vi "Caller VI_ApplyLibIconOverlayToVIIcon.vi"(4 "External User Layer":refnum<class "Layer.lvclass">[](array[class]), 6 "Add Ext User Layer? (F)":bool, 7 "Lib Refnum":refnum<vi>, 8 "Don't Consider Curr VI Icon? (F)":bool, 9 "Overlay Image":T1={"image type"=0, "image depth"=0, "image"=[], "mask"=[], "colors"=[], "Rectangle"={"left"=0, "top"=0, "right"=32, "bottom"=32}}, 10 "Overlay Provided?":bool, 11 "VI Refnum":refnum<vi>) -> (0 "Error Code Out":i32)   [LabVIEW 2021]
uses:
  <vilib>/picture/picture.llb/imagedata.ctl
  vi.lib/LabVIEW Icon API/lv_icon/Classes/Layer/Layer.lvclass
  vi.lib/LabVIEW Icon API/lv_icon/Classes/Icon/Icon.lvclass
  TypeDefs/Cluster_Layer Data.ctl
  TypeDefs/Cluster_Path&Icon.ctl
  vi.lib/LabVIEW Icon API/lv_icon/lv_icon.lvlib
  vi.lib/LabVIEW Icon API/lv_icon/Classes/Icon Framework/Icon Framework.lvclass
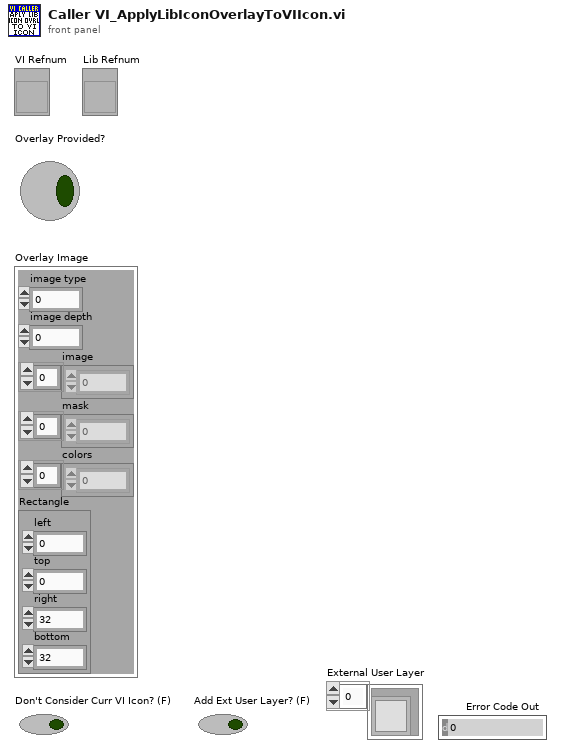
[diagram p1: front panel]
types:
  T1 = typedef "imagedata.ctl" = cluster{"image type":i32, "image depth":i32, "image":u8[], "mask":u8[], "colors":u32[], "Rectangle":cluster{"left":i16, "top":i16, "right":i16, "bottom":i16}}
  T2 = typedef "Cluster_Path&Icon.ctl" = cluster{"Rectangle":cluster{"left":i16, "top":i16, "right":i16, "bottom":i16}, "Path":path, "Image":picture, "Filter":string, "FileName":string}
  T3 = typedef "Cluster_Layer Data.ctl" = cluster{"LayerIcon":picture, "LayerName":string, "Opacity":u8, "Visibility?":bool}
  T4 = typedef "Cluster_INI Data.ctl" = cluster{"Show Layer Tab?":bool, "Show Terminals?":bool, "Text":cluster{"Font":T5, "Alignment":T6, "Size":T7}, "3rd party Templates":cluster{"Store 3rd party Templates?":bool, "Folder Name":string}, "Merge user layers on commit":bool, "Body Text":T8, "Fill Color":T9, "Edge Color":T9, "Tab":u16, "Tool":T10, "Disable Layers?":bool}
  T5 = typedef "Font.ctl" = string
  T6 = typedef "Alignment.ctl" = u16
  T7 = typedef "Num_Font Size.ctl" = u8
  T8 = typedef "Cluster_BodyText.ctl" = cluster{"Line 1 text":string, "Line 2 text":string, "Line 3 text":string, "Line 4 text":string, "Line 1 color":u32, "Line 2 color":u32, "Line 3 color":u32, "Line 4 color":u32, "Body Text Spec":cluster{"Font":T5, "Alignment":T6, "Size":u8}, "Center text vertically":bool, "Capitalize Text":bool}
  T9 = typedef "IEColor.ctl" = u32
  T10 = typedef "Cluster_Button Draw Tools.ctl" = enum32{"Pencil", "Line", "Dropper", "Fill", "Rectangle", "Filled Rectangle", "Ellipse", "Filled Ellipse", "Eraser", "Text", "Select", "Move"}
  T11 = typedef "LabVIEW Icon Stored Information.ctl" = cluster{"Text Visible?":bool, "Text Opacity":u8, "Templ Visible?":bool, "Templ Opacity":u8, "Relative Path from 1 to 2":path, "Image":picture, "All User Layers":refnum<class "Layer.lvclass">[], "Body Text":T8}
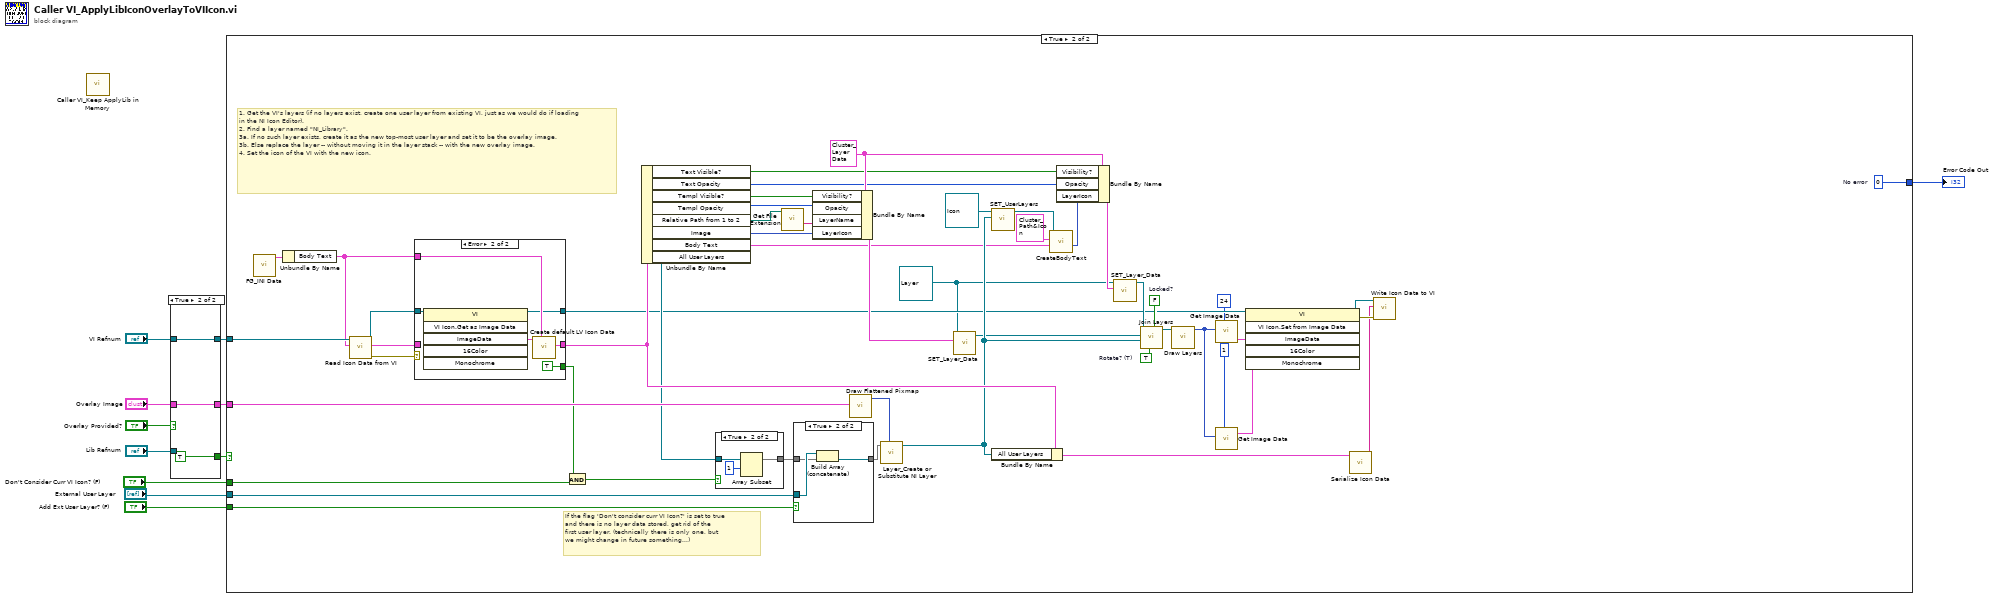
[diagram p0: block diagram]
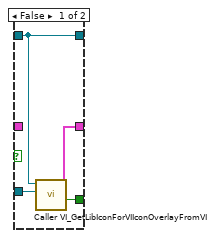
[diagram p2: hidden frame]
diagram:
  n1 = call "Caller VI_Keep ApplyLib in Memory.vi"() -> ()  [unwired: 1 out]
  n2 = case shown="True" "Overlay Provided?" {
    tunnel: "VI Refnum" -> [w12 w16]
    tunnel: [w15 TRUE ("Owned by library?")] -> w11
    tunnel: [w14 w18] -> w10
    tunnel: "Overlay Image" -> [_ w18]
    tunnel: "Lib Refnum" -> [w13 _]
    tunnel: [w12 w16] -> w1
    frame False {
      n3 = call "Caller VI_GetLibIconForVIIconOverlayFromVI.vi"("Lib Refnum"=w13, "VI Refnum"=w12) -> ("Owned by library?"=w15:bool, "Library Icon For VI Overlay"=w14:T1)  [unwired: 8 out]
    }
    frame True {
    }
  }
  n4 = case shown="True" w11 {
    tunnel: w10 -> [_ w67]
    tunnel: [_ w68] -> w7
    tunnel: w1 -> [_ w34]
    tunnel: "Add Ext User Layer? (F)" -> [_ w47]
    tunnel: "External User Layer" -> [_ w46]
    tunnel: "Don't Consider Curr VI Icon? (F)" -> [_ w45]
    frame False {
      # "No work needs to be done. VI is not owned by a library."
    }
    frame True {
      w29 = TRUE  # Rotate? (T)
      w30 = FALSE  # Locked?
      w50 = T3 {"LayerIcon"=bytes[3102], "LayerName"="", "Opacity"=100, "Visibility?"=TRUE} ("Data")
      w19 = refnum<class "Layer.lvclass"> refnum ("Layer.lvclass in")
      w68 = 0  # No error
      # "If the flag 'Don't consider curr VI Icon?' is set to true\nand there is no layer data stored, get rid of the\nfirst user layer. (technically there is only one, but\nwe might change in future something...)"
      # "1. Get the VI's layers (if no layers exist, create one user layer from existing VI, just as we would do if loading in the NI Icon Editor).\n2. Find a layer named \"NI_Library\".\n3a. If no such layer exists, create it as the new top-most user layer and set it to be the overlay image.\n3b. Else replace the layer -- without moving it in the layer stack -- with the new overlay image.\n4. Set the icon of the VI with the new icon."
      n5 = call "FG_INI Data.vi"() -> ("INI Data Out"=w40:T4)  [unwired: 1 in, 10 out]
      n6 = Unbundle By Name(w40) -> ("Body Text"=w32:T8)
      n7 = call "Read Icon Data from VI.vi"("Default body text"=w32, "VI Ref in"=w34) -> ("error out"=w31:errorcluster, "Data"=w33:T11, "VI Ref out"=w27:refnum<vi>)  [unwired: 7 in]
      n8 = case shown="Error" w31 {
        tunnel: w33 -> [w78 _]
        tunnel: [w78 w81] -> w63
        tunnel: w27 -> [w77 w84]
        tunnel: [_ TRUE] -> w44
        tunnel: w32 -> [_ w80]
        tunnel: [w77 w79] -> w26
        frame No Error {
        }
        frame Error {
          n9 = invoke class="VI" method="VI Icon.Get as Image Data"(reference=w84) -> (reference out=w79:refnum<vi>, "ImageData"=w82:T1)  [unwired: 5 in, 4 out]
          n10 = call "Create default LV Icon Data.vi"("Body Text"=w80, "Pic Data"=w82) -> ("VI Icon Data Out"=w81:T11)  [unwired: 8 in, 1 out]
        }
      }
      n11 = And(x=w44, y=w45) -> (x .and. y?=w42:bool)
      n12 = Unbundle By Name(w63) -> ("Text Visible?"=w20:bool, "Text Opacity"=w21:u8, "Templ Visible?"=w62:bool, "Templ Opacity"=w61:u8, "Relative Path from 1 to 2"=w60:path, "Image"=w58:picture, "Body Text"=w22:T8, "All User Layers"=w43:refnum<class "Layer.lvclass">[])
      n13 = case shown="True" w42 {
        tunnel: w43 -> [w69 w72]
        tunnel: [w69 w70] -> w41
        frame False {
        }
        frame True {
          n14 = Array Subset(array=w72, index=1) -> (w70:refnum<class "Layer.lvclass">[])  [unwired: 1 in]
        }
      }
      n15 = call <vilib>:"Get File Extension.vi"("file"=w60) -> ("filename without extension"=w59:string)  [unwired: 6 in, 4 out]
      n16 = case shown="True" w47 {
        tunnel: w41 -> [w73 w75]
        tunnel: [w73 w74] -> w48
        tunnel: w46 -> [_ w76]
        frame False {
        }
        frame True {
          n17 = Build Array (concatenate)(w76, w75) -> (w74:refnum<class "Layer.lvclass">[])
        }
      }
      n18 = Bundle By Name(cluster=w50, "Visibility?"=w62, "Opacity"=w61, "LayerName"=w59, "LayerIcon"=w58) -> (w55:T3)
      n19 = call <vilib>:"Draw Flattened Pixmap.vi"("image data"=w67) -> ("new picture"=w28:picture)  [unwired: 1 in, 7 out]
      n20 = call "Layer_Create or Substitute NI Layer.vi"("New Picture"=w28, "All Layers"=w48) -> ("All Layers Out"=w56:refnum<class "Layer.lvclass">[])  [unwired: 9 in]
      n21 = call-dynamic "SET_Layer_Data.vi"("Data"=w55, "Layer.lvclass in"=w19) -> ("Layer.lvclass out"=w54:refnum<class "Layer.lvclass">)  [unwired: 8 in, 1 out]
      n22 = call-dynamic "SET_UserLayers.vi"("Layers"=w56, "Icon.lvclass in"=refnum<class "Icon.lvclass"> refnum) -> ("Icon.lvclass out"=w39:refnum<class "Icon.lvclass">)  [unwired: 8 in, 1 out]
      n23 = Bundle By Name(cluster=w63, "All User Layers"=w56) -> (w38:T11)
      n24 = call "CreateBodyText.vi"("Body Text"=w22, "Path And Icon"=T2 {"Rectangle"={"left"=0, "top"=0, "right"=0, "bottom"=0}, "Path"=path "", "Image"=bytes[0], "Filter"="", "FileName"=""} ("Path and Icon Template"), "Icon.lvclass"=w39) -> ("Body Text Out"=w23:picture)  [unwired: 1 in, 7 out]
      n25 = Bundle By Name(cluster=w50, "Visibility?"=w20, "Opacity"=w21, "LayerIcon"=w23) -> (w51:T3)
      n26 = call-dynamic "SET_Layer_Data.vi"("Data"=w51, "Layer.lvclass in"=w19) -> ("Layer.lvclass out"=w49:refnum<class "Layer.lvclass">)  [unwired: 8 in, 1 out]
      n27 = call "Join Layers.vi"("Locked?"=w30, "Rotate? (T)"=w29, "User Layers"=w56, "Template"=w54, "Icon Text"=w49) -> ("Layer Out"=w53:refnum<class "Layer.lvclass">[])  [unwired: 1 in, 5 out]
      n28 = call "Draw Layers.vi"("Layers"=w53) -> ("Picture"=w52:picture)  [unwired: 4 in, 6 out]
      n29 = call "Get Image Data.vi"("Depth (24)"=24, "Pic"=w52) -> ("Image Data Out"=w65:T1)  [unwired: 2 in, 7 out]
      n30 = call "Get Image Data.vi"("Depth (24)"=1 ("depth"), "Pic"=w52) -> ("Image Data Out"=w64:T1)  [unwired: 2 in, 7 out]
      n31 = invoke class="VI" method="VI Icon.Set from Image Data"(reference=w26, "ImageData"=w65, "Monochrome"=w64) -> (reference out=w35:refnum<vi>, error out=w37:errorcluster)  [unwired: 3 in, 4 out]
      n32 = call "Serialize Icon Data.vi"("Icon data"=w38) -> ("data string"=w36:string)  [unwired: 9 in, 1 out]
      n33 = call "Write Icon Data to VI.vi"("error in (no error)"=w37, "Data"=w36, "VI Ref in"=w35) -> ()  [unwired: 7 in, 2 out]
    }
  }
  "Error Code Out" <- w7
